vi "Control MagnaDC via ADAM Table.vi"() -> ()   [LabVIEW 2021]
doc: "Simple example how to control power supplu output using voltage and current levels."
uses:
  Anemometry/Anemometry Sub Vis/Globals/Preference_global.vi
  Magna sub vis/MagnaDC.lvlib
panel:
  in  "Limit":dbl[](array[numeric])=[4000.0, 1000.0, 250.0, 100.0, 8.0, 80.0, 60.0]
  out "Monitored channels":string[](array[string])
  out "Value":dbl[](array[numeric]) format="%#.2g"
  in  "Aero_Tunnel:EDF:Dem RPM":dbl=5.0
  in  "Press to set  rpm":bool
  in  "DC:Supply:Dem Volts":dbl=5.0 format="%.2f"
  in  "Press to set Volts":bool
  out "Demanded Volts":dbl=5.0 format="%.2f"
  out "ADAM Ch  DC:Supply:Dem Volts":dbl=5.0 format="%.2f"
  out "OCP Tripped":bool
  out "OVP Tripped":bool
  out "Current (A)":dbl=0.2
  out "Voltage (V)":dbl=203.0
  in  "Stop":bool
  in  "Set Current Limit (A)":dbl=15.0 format="%.2f"
  out "error out":errorcluster
  in  "error in (no error)":errorcluster
  in  "VISA resource name":refnum<visa-resource-name>="TCPIP0::131.227.181.163::50505::SOCKET"
  # "Output Values"
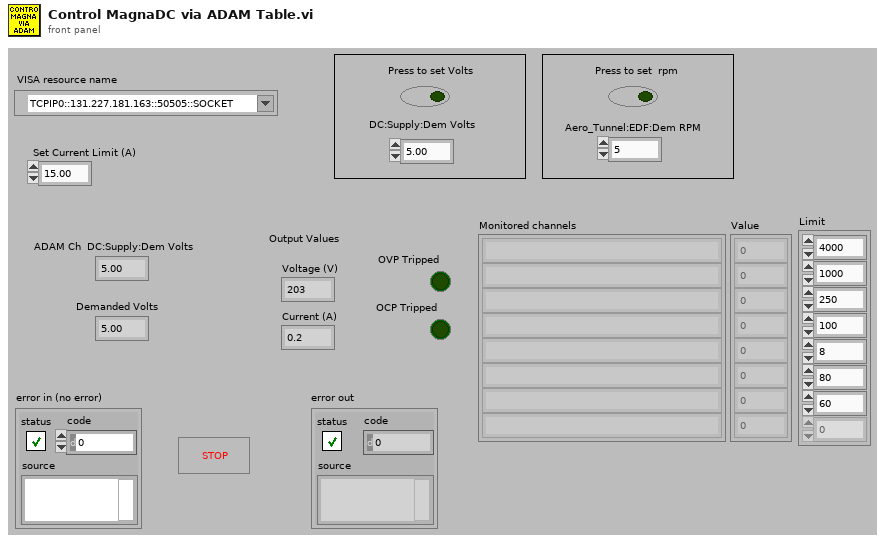
[diagram p1: front panel]
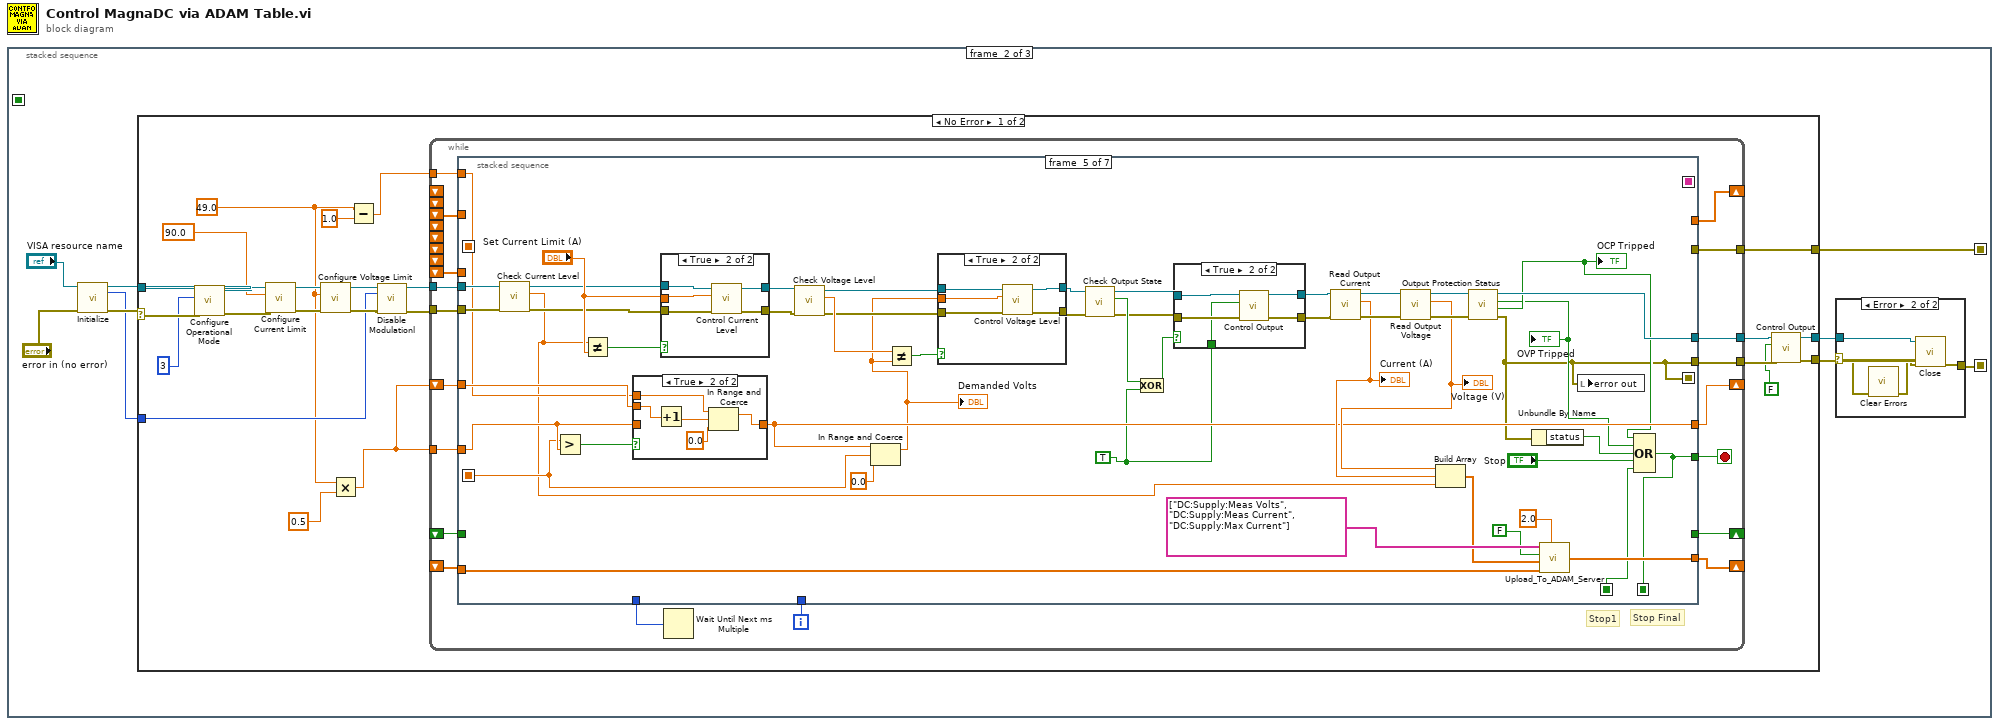
[diagram p0: block diagram]
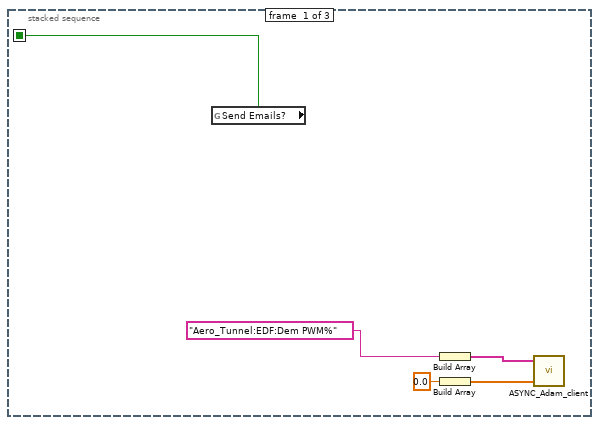
[diagram p2: hidden frame]
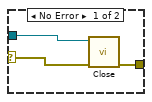
[diagram p3: hidden frame]
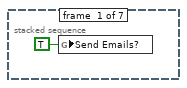
[diagram p4: hidden frame]
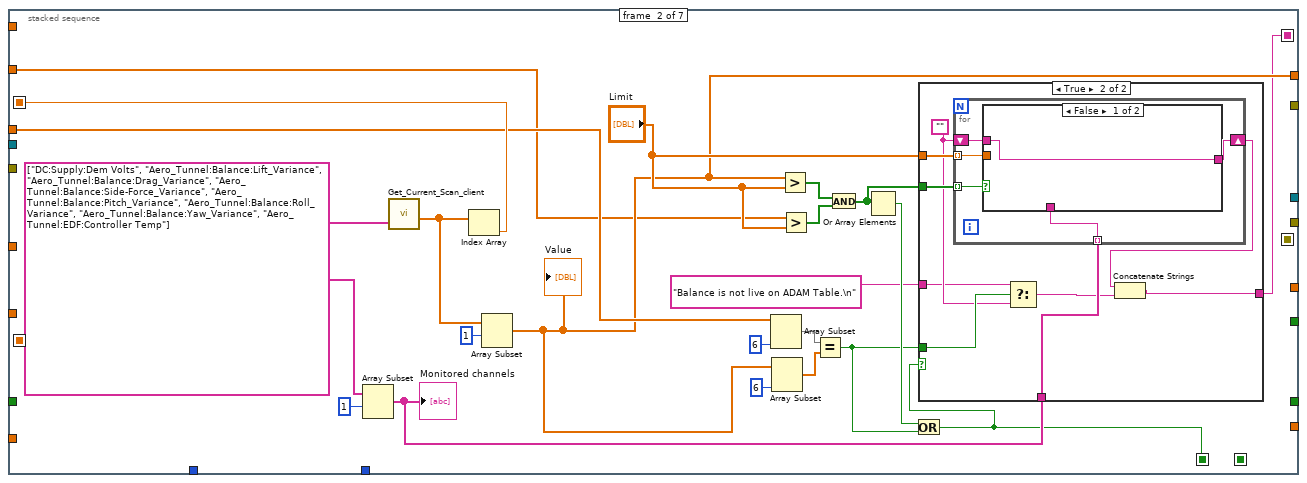
[diagram p5: hidden frame]
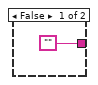
[diagram p6: hidden frame]
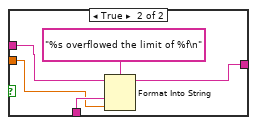
[diagram p7: hidden frame]
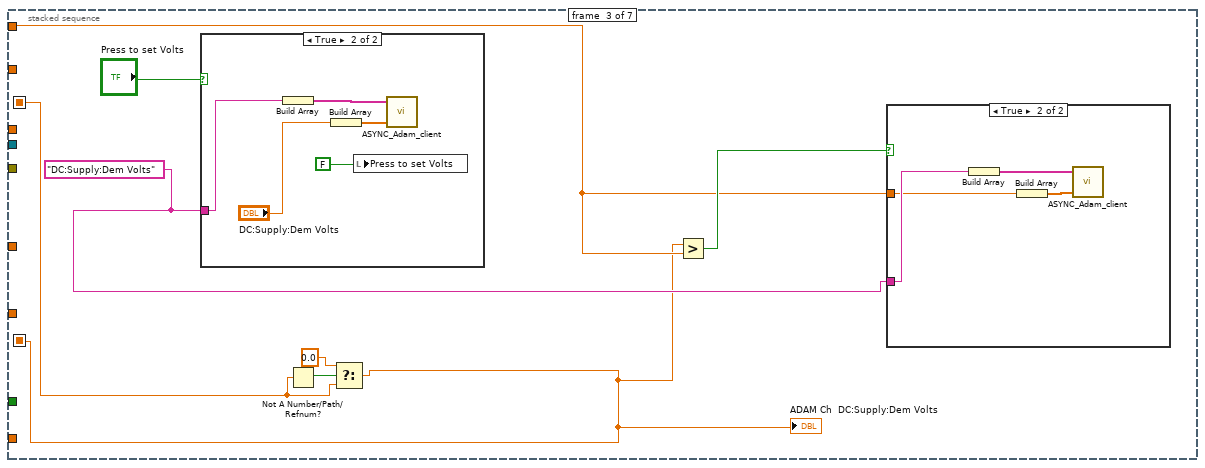
[diagram p8: hidden frame]
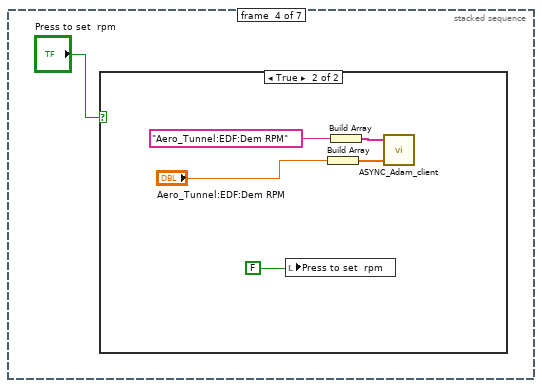
[diagram p11: hidden frame]
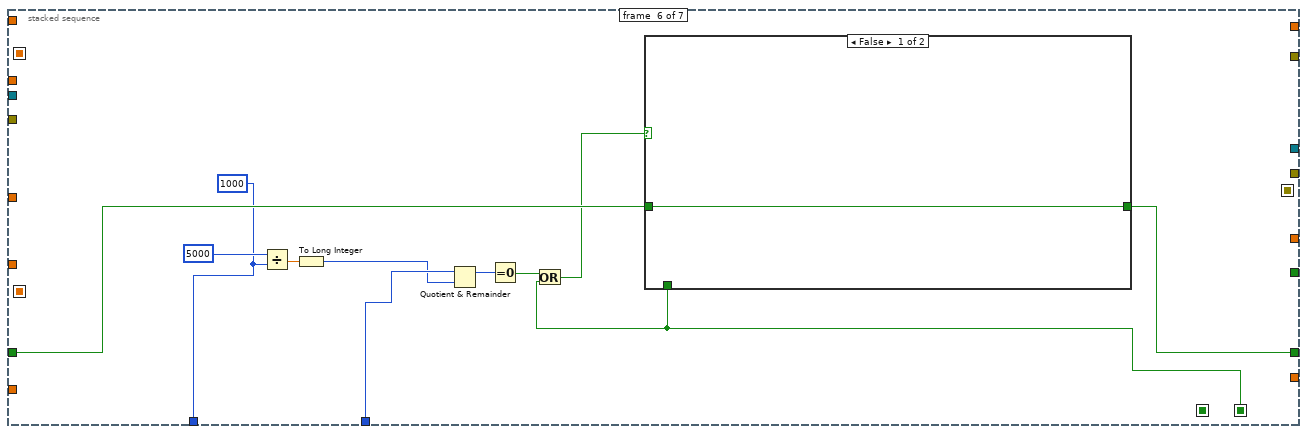
[diagram p17: hidden frame]
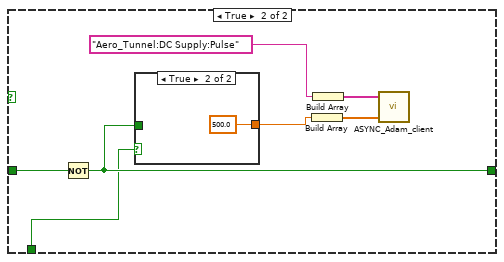
[diagram p18: hidden frame]
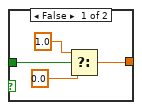
[diagram p19: hidden frame]
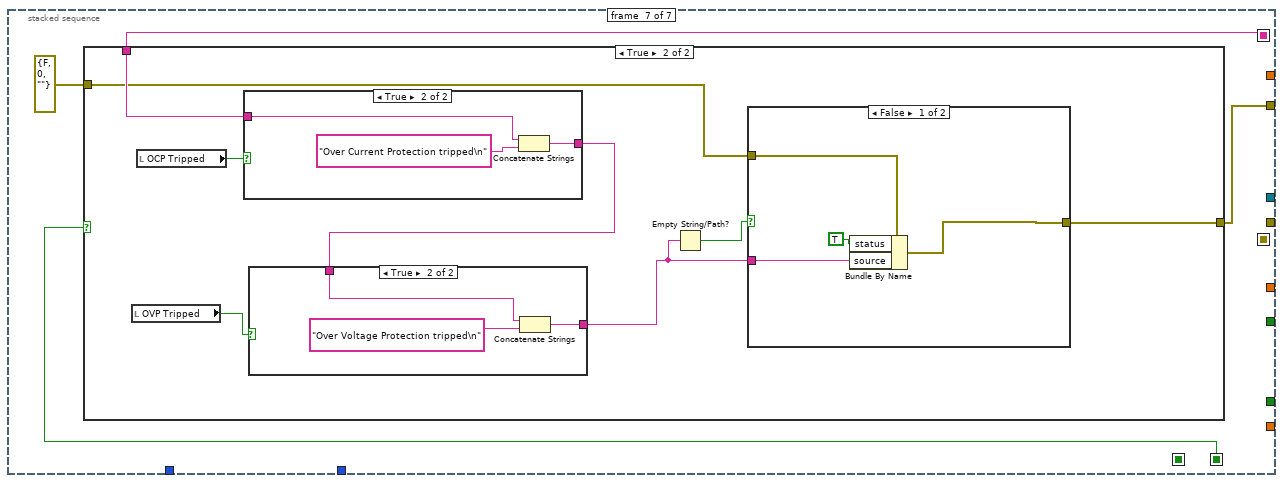
[diagram p20: hidden frame]
diagram:
  n1 = stacked-sequence {
    seq-local: [w5 _ _] -> [_ _ w273]
    seq-local: [_ w7 _] -> [_ _ w262]
    seq-local: [_ w6 _] -> [_ _ w263]
    frame #0 {
      n2 = global read "Preference_global.vi" "Send Emails?"() -> (w5:bool)
      n3 = Build Array("Aero_Tunnel:EDF:Dem PWM%") -> (w4:string[])
      n4 = Build Array(0.0 ("element")) -> (w3:dbl[])
      n5 = call "ASYNC_Adam_client.vi"("Values"=w3, "Channel Names"=w4) -> ()  [unwired: 1 in, 2 out]
    }
    frame #1 {
      n6 = call "Initialize.vi"("VISA resource name"="VISA resource name", "error in (no error)"="error in (no error)") -> ("VISA resource name out"=w12:refnum<visa-resource-name>, "Modulation Available"=w9:u32, "error out"=w13:errorcluster)  [unwired: 10 in, 1 out]
      n7 = case shown="No Error" w13 {
        selector: w13 -> [w44 w259]
        tunnel: w12 -> [w45 w260]
        tunnel: [w23 w259] -> w11
        tunnel: [w42 w260] -> w10
        tunnel: w9 -> [w30 _]
        tunnel: [w22 w259] -> w6
        frame No Error {
          w26 = 49.0 ("OVP (V)")
          n8 = call "Configure Operational Mode.vi"("error in (no error)"=w44, "Operational Mode"=u32 3, "VISA resource name"=w45) -> ("error out"=w36:errorcluster, "VISA resource name out"=w38:refnum<visa-resource-name>)  [unwired: 7 in]
          n9 = call "Configure Current Limit.vi"("error in (no error)"=w36, "Current Limit (0.0 A)"=90.0 ("OCP (A)"), "VISA resource name"=w38) -> ("error out"=w35:errorcluster, "VISA resource name out"=w37:refnum<visa-resource-name>)  [unwired: 7 in]
          n10 = call "Configure Voltage Limit.vi"("error in (no error)"=w35, "Voltage Limit (0.0 V)"=w26, "VISA resource name"=w37) -> ("error out"=w34:errorcluster, "VISA resource name out"=w33:refnum<visa-resource-name>)  [unwired: 7 in]
          n11 = Multiply(x=w26, y=0.5) -> (x*y=w24:dbl)
          n12 = Subtract(x=w26, y=1.0) -> (x-y=w27:dbl)
          n13 = call "Disable Modulationl.vi"("VISA resource name"=w33, "Modulation"=w30, "error in (no error)"=w34) -> ("VISA resource name out"=w32:refnum<visa-resource-name>, "error out"=w31:errorcluster)  [unwired: 11 in]
          n14 = while {
            tunnel: [w58] -> w40
            tunnel: [w63] -> w41
            tunnel: w32 -> [w62]
            tunnel: w31 -> [w61]
            shift-right: [w59] -> _
            shift-left: _ -> [w60]
            shift-right: [w54] -> _
            shift-left: w24 -> [w56]
            tunnel: w27 -> [w55]
            tunnel: w24 -> [w57]
            shift-right: [w53] -> _
            shift-left: _ -> [_]
            shift-left: _ -> [_]
            shift-left: _ -> [w48]
            shift-right: [w51] -> _
            shift-left: _ -> [w50]
            shift-left: _ -> [_]
            shift-left: _ -> [_]
            shift-left: _ -> [_]
            shift-left: _ -> [_]
            shift-left: _ -> [w49]
            tunnel: [w46] -> w22
            i -> [w52]
            stop <- w64 stop-if-true
            # "Stop Final"
            # "Stop1"
            n15 = stacked-sequence {
              seq-local: [_ _ w109 _ _ _ _] -> [_ _ _ _ w138 _ _]
              seq-local: [_ w87 _ _ _ _ _] -> [_ _ w112 _ _ _ _]
              seq-local: [_ w70 _ _ _ _ _] -> [_ _ _ _ w137 _ _]
              seq-local: [_ _ _ _ w133 _ _] -> [_ _ _ _ _ w209 w236]
              seq-local: [_ w66 _ _ _ _ _] -> [_ _ _ _ _ _ w235]
              seq-local: [_ _ _ _ w132 _ _] -> [_ _ _ _ _ _ _]
              tunnel: [_ _ _ _ w133 _ _] -> w64
              tunnel: [_ _ _ _ w175 _ _] -> w63
              tunnel: w62 -> [_ _ _ _ w156 _ _]
              tunnel: w61 -> [_ _ _ _ w155 _ _]
              tunnel: w60 -> [_ _ _ _ w151 _ _]
              tunnel: [_ _ _ _ w150 _ _] -> w59
              tunnel: [_ _ _ _ w132 _ _] -> w58
              tunnel: w57 -> [_ _ _ _ w145 _ _]
              tunnel: w56 -> [_ _ _ _ w144 _ _]
              tunnel: w55 -> [_ _ w110 _ w143 _ _]
              tunnel: [_ _ _ _ w142 _ _] -> w54
              tunnel: [_ w73 _ _ _ _ _] -> w53
              tunnel: w49 -> [_ w75 _ _ _ _ _]
              tunnel: w52 -> [_ _ _ _ _ w219 _]
              tunnel: [_ _ _ _ _ w215 _] -> w51
              tunnel: w50 -> [_ _ _ _ _ w214 _]
              tunnel: w48 -> [_ w67 _ _ _ _ _]
              tunnel: [_ _ _ _ _ w213 _] -> w47
              tunnel: [_ _ _ _ _ _ w234] -> w46
              frame #0 {
                n16 = global write "Preference_global.vi" "Send Emails?"(TRUE ("Send Emails?")) -> ()
              }
              frame #1 {
                w83 = string[] ["DC:Supply:Dem Volts", "Aero_Tunnel:Balance:Lift_Variance", "Aero_Tunnel:Balance:Drag_Variance", "Aero_Tunnel:Balance:Side-Force_Variance", "Aero_Tunnel:Balance:Pitch_Variance", "Aero_Tunnel:Balance:Roll_Variance", "Aero_Tunnel:Balance:Yaw_Variance", "Aero_Tunnel:EDF:Controller Temp"]
                n17 = Array Subset(array=w83, index=1) -> (w77:string[])  [unwired: 1 in]
                "Monitored channels" <- w77
                n18 = call "Get_Current_Scan_client.vi"("multipleChannels"=w83) -> ("Numerical Values"=w86:dbl[])  [unwired: 1 in, 3 out]
                n19 = Index Array(array=w86) -> (element=w87:dbl)  [unwired: 1 in]
                n20 = Array Subset(array=w86, index=1) -> (w73:dbl[])  [unwired: 1 in]
                "Value" <- w73
                n21 = Array Subset(array=w75, length=6) -> (w72:dbl[])  [unwired: 1 in]
                n22 = Array Subset(array=w73, length=6) -> (w71:dbl[])  [unwired: 1 in]
                n23 = Greater?(x=w73, y="Limit") -> (0:w82:bool[])
                n24 = Greater?(x=w67, y="Limit") -> (0:w81:bool[])
                n25 = Equal?(x=w72, y=w71) -> (x = y?=w69:bool)
                n26 = And(x=w82, y=w81) -> (x .and. y?=w80:bool[])
                n27 = Or Array Elements(Boolean array=w80) -> (logical OR=w79:bool)
                n28 = Or(x=w79, y=w69) -> (x .or. y?=w70:bool)
                n29 = case shown="True" w70 {
                  tunnel: w80 -> [_ w97]
                  tunnel: "Limit" -> [_ w96]
                  tunnel: w77 -> [_ w95]
                  tunnel: w69 -> [_ w93]
                  tunnel: "Balance is not live on ADAM Table.\n" ("t") -> [_ w90]
                  tunnel: ["" w89] -> w66
                  frame False {
                  }
                  frame True {
                    w92 = ""
                    n30 = for {
                      tunnel: w97 -> [w102] mode=indexing
                      tunnel: w96 -> [w101] mode=indexing
                      tunnel: w95 -> [w100] mode=indexing
                      shift-right: [w98] -> w94
                      shift-left: w92 -> [w99]
                      n31 = case shown="False" w102 {
                        tunnel: w101 -> [_ w107]
                        tunnel: w100 -> [_ w108]
                        tunnel: w99 -> [w103 w106]
                        tunnel: [w103 w105] -> w98
                        frame False {
                        }
                        frame True {
                          n32 = Format Into String(format string="%s overflowed the limit of %f\n", initial string=w106, w108, w107) -> (resulting string=w105:string)  [unwired: 1 in, 1 out]
                        }
                      }
                    }
                    n33 = Select(t=w90, s=w93, f=w92) -> (s? t:f=w91:string)
                    n34 = Concatenate Strings(w94, w91) -> (w89:string)
                  }
                }
              }
              frame #2 {
                w111 = "DC:Supply:Dem Volts"
                n35 = case shown="True" "Press to set Volts" {
                  tunnel: w111 -> [_ w124]
                  frame False {
                  }
                  frame True {
                    n36 = Build Array(w124) -> (w125:string[])
                    n37 = Build Array("DC:Supply:Dem Volts") -> (w123:dbl[])
                    n38 = local write "Press to set Volts"(FALSE ("Press to set")) -> ()
                    n39 = call "ASYNC_Adam_client.vi"("Values"=w123, "Channel Names"=w125) -> ()  [unwired: 1 in, 2 out]
                  }
                }
                n40 = Not A Number/Path/Refnum?(number/path/refnum=w112) -> (NaN/Path/Refnum?=w116:bool)
                n41 = Select(t=0.0, s=w116, f=w112) -> (s? t:f=w109:dbl)
                "ADAM Ch  DC:Supply:Dem Volts" <- w109
                n42 = Greater?(x=w109, y=w110) -> (0:w113:bool)
                n43 = case shown="True" w113 {
                  tunnel: w111 -> [_ w119]
                  tunnel: w110 -> [_ w117]
                  frame False {
                  }
                  frame True {
                    n44 = Build Array(w119) -> (w120:string[])
                    n45 = Build Array(w117) -> (w118:dbl[])
                    n46 = call "ASYNC_Adam_client.vi"("Values"=w118, "Channel Names"=w120) -> ()  [unwired: 1 in, 2 out]
                  }
                }
              }
              frame #3 {
                n47 = case shown="True" "Press to set  rpm" {
                  frame False {
                  }
                  frame True {
                    n48 = local write "Press to set  rpm"(FALSE ("Press to set")) -> ()
                    n49 = Build Array("Aero_Tunnel:EDF:Dem RPM") -> (w130:dbl[])
                    n50 = Build Array("Aero_Tunnel:EDF:Dem RPM" ("String")) -> (w131:string[])
                    n51 = call "ASYNC_Adam_client.vi"("Values"=w130, "Channel Names"=w131) -> ()  [unwired: 1 in, 2 out]
                  }
                }
              }
              frame #4 {
                w139 = TRUE ("Output")
                n52 = call "Check Current Level.vi"("error in (no error)"=w155, "VISA resource name"=w156) -> ("error out"=w160:errorcluster, "Current Level (A)"=w136:dbl, "VISA resource name out"=w159:refnum<visa-resource-name>)  [unwired: 7 in]
                n53 = Greater?(x=w138, y=w145) -> (0:w146:bool)
                n54 = Not Equal?(x=w136, y="Set Current Limit (A)") -> (x != y?=w161:bool)
                n55 = case shown="True" w146 {
                  tunnel: [w182 w185] -> w142
                  tunnel: w145 -> [w182 _]
                  tunnel: w144 -> [_ w187]
                  tunnel: w143 -> [_ w183]
                  frame False {
                  }
                  frame True {
                    n56 = Increment(x=w187) -> (x+1=w184:dbl)
                    n57 = In Range and Coerce(upper limit=w183, x=w184, lower limit=0.0) -> (coerced(x)=w185:dbl)  [unwired: 1 out]
                  }
                }
                n58 = case shown="True" w161 {
                  tunnel: w160 -> [w195 w201]
                  tunnel: w159 -> [w196 w200]
                  tunnel: [w196 w199] -> w165
                  tunnel: [w195 w198] -> w166
                  tunnel: "Set Current Limit (A)" -> [_ w197]
                  frame False {
                  }
                  frame True {
                    n59 = call "Control Current Level.vi"("error in (no error)"=w201, "Current Level (0.0 A)"=w197, "VISA resource name"=w200) -> ("error out"=w198:errorcluster, "VISA resource name out"=w199:refnum<visa-resource-name>)  [unwired: 7 in]
                  }
                }
                n60 = call "Check Voltage Level.vi"("error in (no error)"=w166, "VISA resource name"=w165) -> ("error out"=w164:errorcluster, "Voltage Level (V)"=w168:dbl, "VISA resource name out"=w163:refnum<visa-resource-name>)  [unwired: 7 in]
                n61 = In Range and Coerce(upper limit=w142, x=w138, lower limit=0.0) -> (coerced(x)=w140:dbl)  [unwired: 1 out]
                "Demanded Volts" <- w140
                n62 = Not Equal?(x=w168, y=w140) -> (x != y?=w167:bool)
                n63 = case shown="True" w167 {
                  tunnel: w163 -> [w189 w194]
                  tunnel: w164 -> [w188 w193]
                  tunnel: [w189 w192] -> w158
                  tunnel: [w188 w191] -> w157
                  tunnel: w140 -> [_ w190]
                  frame False {
                  }
                  frame True {
                    n64 = call "Control Voltage Level.vi"("error in (no error)"=w193, "Voltage Level (0.0 V)"=w190, "VISA resource name"=w194) -> ("error out"=w191:errorcluster, "VISA resource name out"=w192:refnum<visa-resource-name>)  [unwired: 7 in]
                  }
                }
                n65 = call "Check Output State.vi"("error in (no error)"=w157, "VISA resource name"=w158) -> ("error out"=w171:errorcluster, "Output"=w174:bool, "VISA resource name out"=w172:refnum<visa-resource-name>)  [unwired: 7 in]
                n66 = Exclusive Or(1:w139, 2:w174) -> (0:w173:bool)
                n67 = case shown="True" w173 {
                  tunnel: w172 -> [w203 w208]
                  tunnel: w171 -> [w202 w207]
                  tunnel: [w203 w206] -> w170
                  tunnel: [w202 w205] -> w169
                  tunnel: w139 -> [_ w204]
                  frame False {
                  }
                  frame True {
                    n68 = call "Control Output.vi"("error in (no error)"=w207, "Enable Output (T: Enable)"=w204, "VISA resource name"=w208) -> ("error out"=w205:errorcluster, "VISA resource name out"=w206:refnum<visa-resource-name>)  [unwired: 7 in]
                  }
                }
                n69 = call "Read Output Current.vi"("error in (no error)"=w169, "VISA resource name"=w170) -> ("error out"=w179:errorcluster, "Actual Current Level (A)"=w149:dbl, "VISA resource name out"=w180:refnum<visa-resource-name>)  [unwired: 6 in]
                "Current (A)" <- w149
                n70 = call "Read Output Voltage.vi"("error in (no error)"=w179, "VISA resource name"=w180) -> ("error out"=w177:errorcluster, "Actual Voltage Level (V)"=w147:dbl, "VISA resource name out"=w178:refnum<visa-resource-name>)  [unwired: 7 in]
                "Voltage (V)" <- w147
                n71 = Build Array(w147, w149, w136) -> (w148:dbl[])
                n72 = call "Output Protection Status.vi"("error in (no error)"=w177, "VISA resource name"=w178) -> ("error out"=w132:errorcluster, "OCP Tripped"=w135:bool, "OVP Tripped"=w134:bool, "VISA resource name out"=w175:refnum<visa-resource-name>)  [unwired: 6 in]
                "OVP Tripped" <- w134
                "OCP Tripped" <- w135
                n73 = Unbundle By Name(w132) -> ("status"=w176:bool)
                n74 = call "Upload_To_ADAM_Server.vi"("Averaging Period (s)"=2.0, "Shift In"=w151, "Channel Values"=w148, "Give Variance"=FALSE, "Channel Names"=string[] ["DC:Supply:Meas Volts", "DC:Supply:Meas Current", "DC:Supply:Max Current"]) -> ("Shift Out"=w150:dbl[])  [unwired: 1 in]
                n75 = local write "error out"(w132) -> ()
                n76 = Compound Arithmetic op=OR(w135, w134, w176, "Stop", w137) -> (w133:bool)
              }
              frame #5 {
                w213 = u32 1000 ("millisecond multiple")
                n77 = Divide(x=u32 5000 ("millisecond multiple"), y=w213) -> (x/y=w217:dbl)
                n78 = To Long Integer(number=w217) -> (32bit integer=w216:i32)
                n79 = Quotient & Remainder(x=w219, y=w216) -> (x-y*floor(x/y)=w212:i32)  [unwired: 1 out]
                n80 = Equal To 0?(x=w212) -> (x = 0?=w211:bool)
                n81 = Or(x=w211, y=w209) -> (x .or. y?=w210:bool)
                n82 = case shown="False" w210 {
                  tunnel: [w220 w223] -> w215
                  tunnel: w214 -> [w220 w224]
                  tunnel: w209 -> [_ w221]
                  frame False {
                  }
                  frame True {
                    n83 = Not(x=w224) -> (.not. x?=w223:bool)
                    n84 = case shown="True" w221 {
                      tunnel: w223 -> [w231 _]
                      tunnel: [w230 500.0 ("f")] -> w222
                      frame False {
                        n85 = Select(t=1.0, s=w231, f=0.0) -> (s? t:f=w230:dbl)
                      }
                      frame True {
                      }
                    }
                    n86 = Build Array(w222) -> (w227:dbl[])
                    n87 = Build Array("Aero_Tunnel:DC Supply:Pulse" ("Desired Ch to Read")) -> (w226:string[])
                    n88 = call "ASYNC_Adam_client.vi"("Values"=w227, "Channel Names"=w226) -> ()  [unwired: 1 in, 2 out]
                  }
                }
              }
              frame #6 {
                n89 = case shown="True" w236 {
                  tunnel: w235 -> [_ w243]
                  tunnel: [w237 w239] -> w234
                  tunnel: errorcluster {"status"=FALSE, "code"=0, "source"=""} ("error in (no error)") -> [w237 w238]
                  frame False {
                  }
                  frame True {
                    n90 = local read "OVP Tripped"() -> (w244:bool)
                    n91 = local read "OCP Tripped"() -> (w245:bool)
                    n92 = case shown="True" w245 {
                      tunnel: w243 -> [w255 w258]
                      tunnel: [w255 w256] -> w242
                      frame False {
                      }
                      frame True {
                        n93 = Concatenate Strings(w258, "Over Current Protection tripped\n") -> (w256:string)
                      }
                    }
                    n94 = case shown="True" w244 {
                      tunnel: w242 -> [w251 w253]
                      tunnel: [w251 w252] -> w241
                      frame False {
                      }
                      frame True {
                        n95 = Concatenate Strings(w253, "Over Voltage Protection tripped\n") -> (w252:string)
                      }
                    }
                    n96 = Empty String/Path?(string/path=w241) -> (empty?=w240:bool)
                    n97 = case shown="False" w240 {
                      tunnel: w241 -> [w248 _]
                      tunnel: [w246 w250] -> w239
                      tunnel: w238 -> [w247 w250]
                      frame False {
                        n98 = Bundle By Name(cluster=w247, "status"=TRUE, "source"=w248) -> (w246:errorcluster)
                      }
                      frame True {
                      }
                    }
                  }
                }
              }
            }
            n99 = Wait Until Next ms Multiple(millisecond multiple=w47) -> ()  [unwired: 1 out]
          }
          n100 = call "Control Output.vi"("error in (no error)"=w40, "Enable Output (T: Enable)"=FALSE, "VISA resource name"=w41) -> ("error out"=w23:errorcluster, "VISA resource name out"=w42:refnum<visa-resource-name>)  [unwired: 7 in]
        }
        frame Error {
        }
      }
      n101 = case shown="Error" w11 {
        selector: w11 -> [w17 w21]
        tunnel: [w15 w19] -> w7
        tunnel: w10 -> [w16 w18]
        frame No Error {
          n102 = call "Close.vi"("error in (no error)"=w17, "VISA resource name"=w16) -> ("error out"=w15:errorcluster)  [unwired: 9 in]
        }
        frame Error {
          n103 = call <vilib>:"Clear Errors.vi"("error in (no error)"=w21) -> ("error out"=w20:errorcluster)  [unwired: 5 in, 1 out]
          n104 = call "Close.vi"("error in (no error)"=w20, "VISA resource name"=w18) -> ("error out"=w19:errorcluster)  [unwired: 9 in]
        }
      }
    }
    frame #2 {
      n105 = global write "Preference_global.vi" "Send Emails?"(w273) -> ()
      n106 = Build Array("Aero_Tunnel:EDF:Dem PWM%") -> (w272:string[])
      n107 = Build Array(0.0 ("element")) -> (w270:dbl[])
      n108 = call "ASYNC_Adam_client.vi"("Values"=w270, "Channel Names"=w272) -> ()  [unwired: 1 in, 2 out]
      n109 = call "Get_Current_Scan_client.vi"("singleChannel"="Aero_Tunnel:EDF_Power:Enable") -> ("Numerical Values"=w267:dbl[])  [unwired: 1 in, 3 out]
      n110 = Index Array(array=w267, index=0) -> (element=w265:dbl)
      n111 = Greater Than 0?(x=w265) -> (x > 0?=w264:bool)
      n112 = Merge Errors(w263, w262) -> (w261:errorcluster)
      "error out" <- w261
      n113 = case shown="True" w264 {
        tunnel: w261 -> [_ w275]
        frame False {
        }
        frame True {
          n114 = call "EnFlo_Error_Handler.vi"("error in (no error)"=w275, "Error Type"="Aero Tunnel DC Power Supply Disabled") -> ()  [unwired: 2 in, 2 out]
        }
      }
    }
  }
